vi "0xE6_Read_all_telemetry_data.vi"(7 "error in":errorcluster, 10 "paramUnicorn":T1={"conParam"={"ReadIntParam"=TRUE, "ReadDescrParam"=FALSE, "ReadFloatParam"=TRUE, "debug"=FALSE, "ReadJSON"=TRUE, "IP_address"="192.168.1.216", "N_attempts"=3, "type_con"=enum."TCP", "MB_address"=1, "VISA"="COM1", "connection ID"=refnum, "nameDevices"="", "timeout"=3000, "port"=2000, "type_version"="0F0C0001", "baud_rate"=115200, "VersionControl"=TRUE, "TCP_conn"=TRUE, "WindowSize"=700}, "Param"={"NumParam"={"NTelem"=201, "NInt"=16, "NFloat"=10, "NTable"=2}, "ParamInt"=[{"ID"="Режим работы", "Num"=0, "Name"="", "Type"="", "Enum"="", "Desc"="", "Unit"="", "Access"="", "FormatStr"="", "Min"=0, "Max"=0}, {"ID"="", "Num"=0, "Name"="", "Type"="", "Enum"="", "Desc"="", "Unit"="", "Access"="", "FormatStr"="", "Min"=0, "Max"=0}, {"ID"="", "Num"=0, "Name"="", "Type"="", "Enum"="", "Desc"="", "Unit"="", "Access"="", "FormatStr"="", "Min"=0, "Max"=0}, {"ID"="", "Num"=0, "Name"="", "Type"="", "Enum"="", "Desc"="", "Unit"="", "Access"="", "FormatStr"="", "Min"=0, "Max"=0}, {"ID"="", "Num"=0, "Name"="", "Type"="", "Enum"="", "Desc"="", "Unit"="", "Access"="", "FormatStr"="", "Min"=0, "Max"=0}, {"ID"="", "Num"=0, "Name"="", "Type"="", "Enum"="", "Desc"="", "Unit"="", "Access"="", "FormatStr"="", "Min"=0, "Max"=0}, {"ID"="ModeWork", "Num"=0, "Name"="", "Type"="", "Enum"="", "Desc"="", "Unit"="", "Access"="", "FormatStr"="", "Min"=0, "Max"=0}], "Telemetry"=[], "Table"=[], "ParamFloat"=[]}}) -> (0 "error out":errorcluster, 1 "Telemetry":sgl[](array[numeric]), 2 "TblTelemetry":string[][](array[string]), 3 "paramUnicorn 2":T1={"conParam"={"ReadIntParam"=TRUE, "ReadDescrParam"=FALSE, "ReadFloatParam"=TRUE, "debug"=FALSE, "ReadJSON"=TRUE, "IP_address"="192.168.1.216", "N_attempts"=3, "type_con"=enum."TCP", "MB_address"=1, "VISA"="COM1", "connection ID"=refnum, "nameDevices"="", "timeout"=3000, "port"=2000, "type_version"="0F0C0001", "baud_rate"=115200, "VersionControl"=TRUE, "TCP_conn"=TRUE, "WindowSize"=700}, "Param"={"NumParam"={"NTelem"=201, "NInt"=16, "NFloat"=10, "NTable"=2}, "ParamInt"=[{"ID"="Режим работы", "Num"=0, "Name"="", "Type"="", "Enum"="", "Desc"="", "Unit"="", "Access"="", "FormatStr"="", "Min"=0, "Max"=0}, {"ID"="", "Num"=0, "Name"="", "Type"="", "Enum"="", "Desc"="", "Unit"="", "Access"="", "FormatStr"="", "Min"=0, "Max"=0}, {"ID"="", "Num"=0, "Name"="", "Type"="", "Enum"="", "Desc"="", "Unit"="", "Access"="", "FormatStr"="", "Min"=0, "Max"=0}, {"ID"="", "Num"=0, "Name"="", "Type"="", "Enum"="", "Desc"="", "Unit"="", "Access"="", "FormatStr"="", "Min"=0, "Max"=0}, {"ID"="", "Num"=0, "Name"="", "Type"="", "Enum"="", "Desc"="", "Unit"="", "Access"="", "FormatStr"="", "Min"=0, "Max"=0}, {"ID"="", "Num"=0, "Name"="", "Type"="", "Enum"="", "Desc"="", "Unit"="", "Access"="", "FormatStr"="", "Min"=0, "Max"=0}, {"ID"="ModeWork", "Num"=0, "Name"="", "Type"="", "Enum"="", "Desc"="", "Unit"="", "Access"="", "FormatStr"="", "Min"=0, "Max"=0}], "Telemetry"=[], "Table"=[], "ParamFloat"=[]}})   [LabVIEW 2017, in "LV_Unicorn.lvlib"]
uses:
  LV_Unicorn.lvlib
  Control/unicorn_Param.ctl
  Control/unicorn_conn.ctl
  Control/unicorn_JSON.ctl
  Control/unicorn_ParamInt.ctl
  Control/unicorn_Telemetry.ctl
  Control/unicorn_Table.ctl
  Control/unicorn_ParamFloat.ctl
panel:
  out "String in":string
  out "String out":string
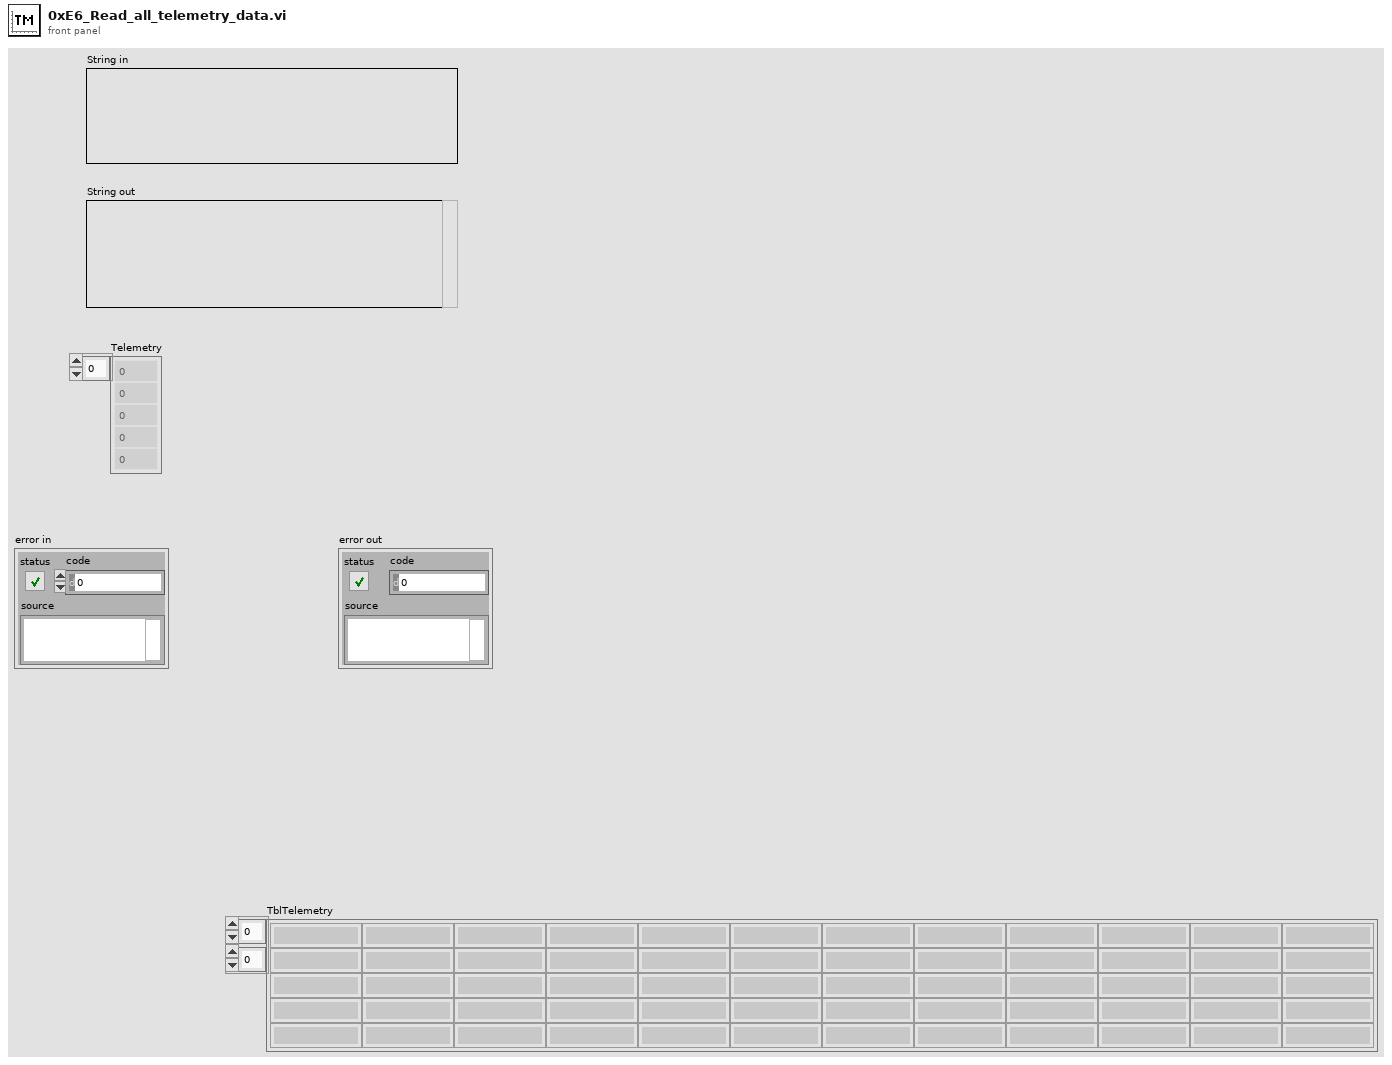
[diagram p1: front panel]
types:
  T1 = typedef "LV_Unicorn.lvlib/unicorn_Param.ctl" = cluster{"conParam":T2, "Param":T3}
  T2 = typedef "LV_Unicorn.lvlib/unicorn_conn.ctl" = cluster{"ReadIntParam":bool, "ReadDescrParam":bool, "ReadFloatParam":bool, "debug":bool, "ReadJSON":bool, "IP_address":string, "N_attempts":i32, "type_con":enum16{"Serial", "TCP"}, "MB_address":i32, "VISA":refnum<visa-resource-name>, "connection ID":refnum<k5>, "nameDevices":string, "timeout":i32, "port":u16, "type_version":string, "baud_rate":u32, "VersionControl":bool, "TCP_conn":bool, "WindowSize":i32}
  T3 = typedef "LV_Unicorn.lvlib/unicorn_JSON.ctl" = cluster{"NumParam":cluster{"NTelem":i32, "NInt":i32, "NFloat":i32, "NTable":i32}, "ParamInt":T4, "Telemetry":T5, "Table":T6, "ParamFloat":T7}
  T4 = typedef "LV_Unicorn.lvlib/unicorn_ParamInt.ctl" = cluster{"ID":string, "Num":i32, "Name":string, "Type":string, "Enum":string, "Desc":string, "Unit":string, "Access":string, "FormatStr":string, "Min":i32, "Max":i32}[]
  T5 = typedef "LV_Unicorn.lvlib/unicorn_Telemetry.ctl" = cluster{"ID":string, "Num":i32, "Name":string, "Desc":string, "Unit":string, "FormatStr":string, "Min":i32, "Max":i32}[]
  T6 = typedef "LV_Unicorn.lvlib/unicorn_Table.ctl" = cluster{"Num":i32, "Access":string, "ColumnCount":i32, "NeedParamPrepare":bool, "Columns":cluster{"Column":i32, "Desc":string, "Name":string}[], "DataType":string, "FormatStr":string, "ID":string, "Name":string, "RowCount":i32, "Rows":cluster{"Desc":string, "ID":string, "Max":i32, "Min":i32, "Name":string, "Row":i32, "Unit":string}[], "Type":string}[]
  T7 = typedef "LV_Unicorn.lvlib/unicorn_ParamFloat.ctl" = cluster{"ID":string, "Num":i32, "Name":string, "Type":string, "Enum":string, "Desc":string, "Unit":string, "Access":string, "FormatStr":string, "Min":sgl, "Max":sgl}[]
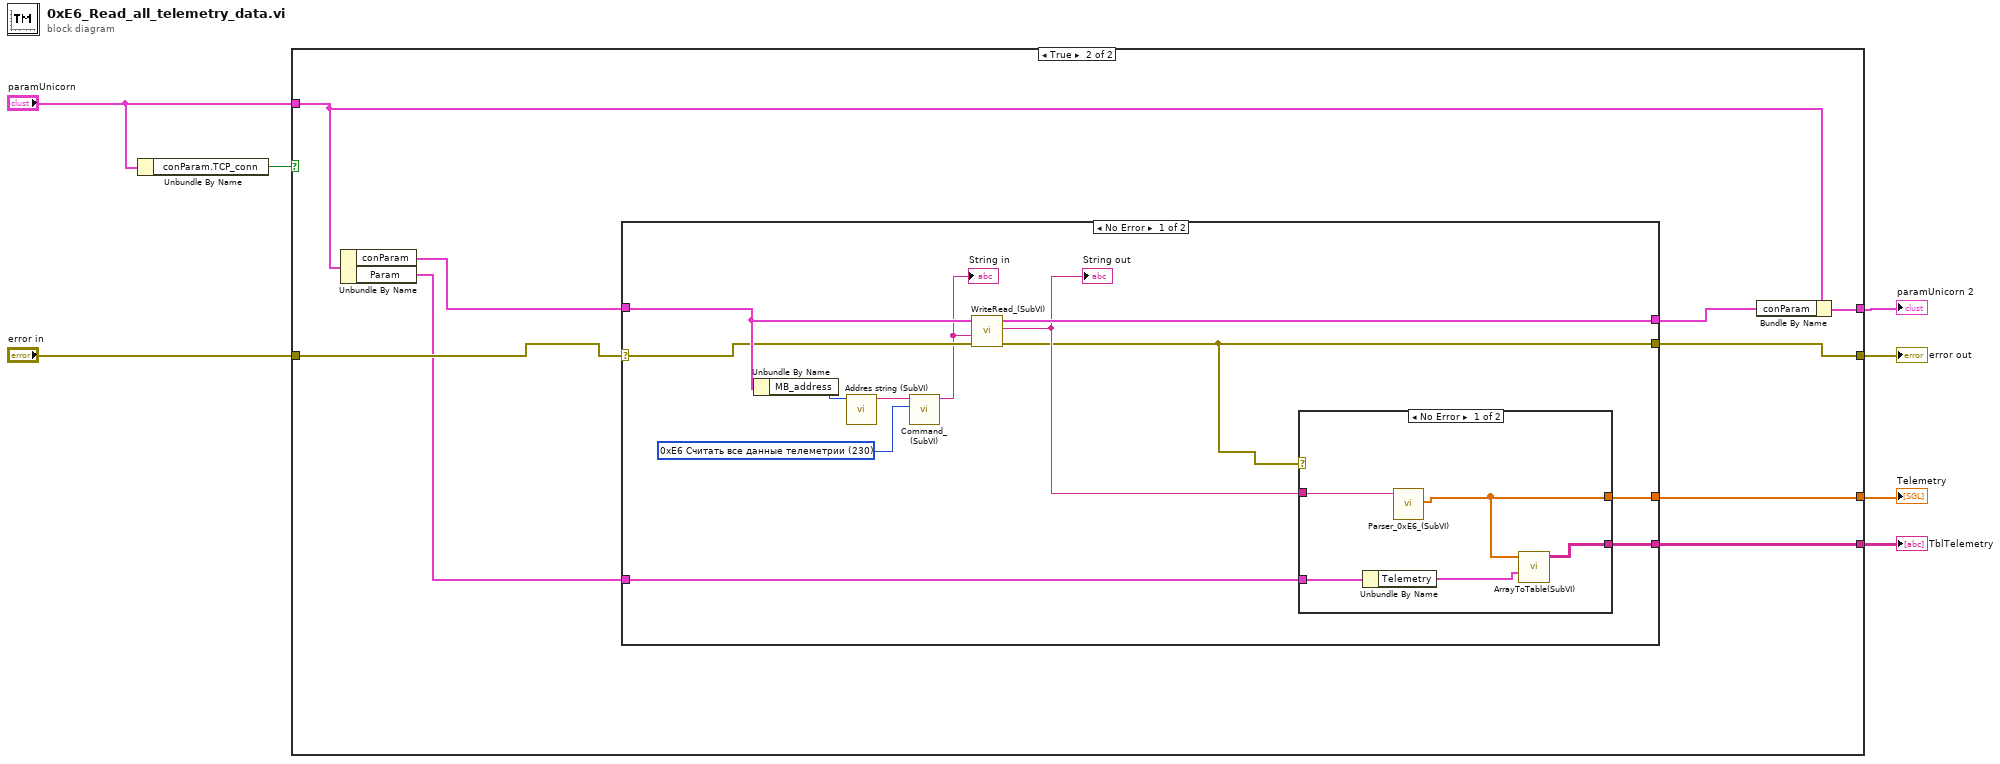
[diagram p0: block diagram]
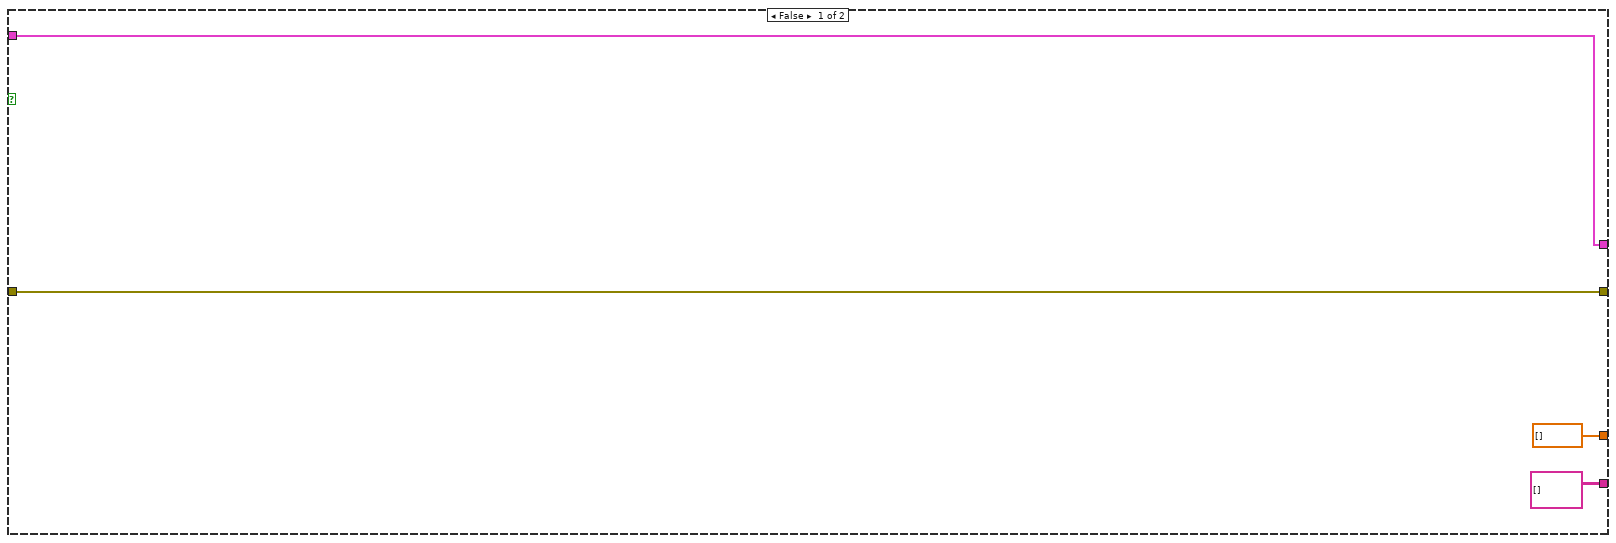
[diagram p2: hidden frame]
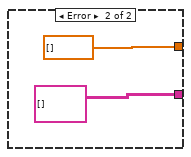
[diagram p3: hidden frame]
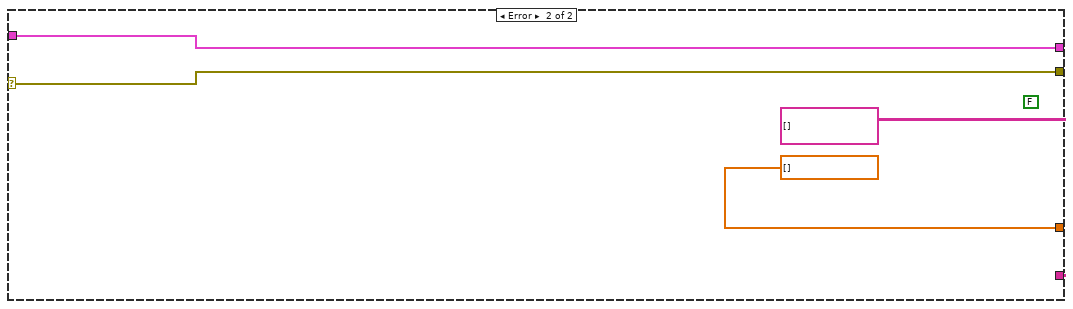
[diagram p4: hidden frame]
diagram:
  n1 = Unbundle By Name("paramUnicorn") -> ("conParam.TCP_conn"=w1:bool)
  n2 = case shown="True" w1 {
    tunnel: [sgl[] [] ("Array") w20] -> w7
    tunnel: "error in" -> [w10 w19]
    tunnel: [w10 w18] -> w5
    tunnel: [string[][] [] ("Таблица телеметрии") w17] -> w4
    tunnel: "paramUnicorn" -> [w11 w14]
    tunnel: [w11 w12] -> w3
    frame False {
    }
    frame True {
      n3 = Unbundle By Name(w14) -> ("conParam"=w16:T2, "Param"=w15:T3)
      n4 = case shown="No Error" w19 {
        selector: w19 -> [w26 w42]
        tunnel: [w32 sgl[] []] -> w20
        tunnel: w16 -> [w27 w43]
        tunnel: [w31 w43] -> w13
        tunnel: [w21 w42] -> w18
        tunnel: [w23 string[][] [] ("Таблица телеметрии")] -> w17
        tunnel: w15 -> [w22 _]
        frame No Error {
          w29 = u16 230 items=["0xE0 Запрос количества доступных параметров"=224, "0xE1 Записать один параметр типа float"=225, "0xE2 Записать один параметр типа int"=226, "0xE3 Считать один параметр телеметрии"=227, "0xE4 Записать все параметры типа float"=228, "0xE5 Записать все параметры типа int"=229, "0xE6 Считать все данные телеметрии"=230, "0xE7 Получить описание одного параметра типа float"=231, "0xE8 Получить описание одного параметра типа int"=232, "0xE9 Получить описание одного параметра телеметрии"=233, "0xEA Считать один параметр типа float"=234, "0xEB Считать один параметр типа int"=235, "0xEC Считать все параметры типа float"=236, "0xED Считать все параметры типа int"=237, "0xEE Считать считать фрагмент описания устройства в формате JSON"=238, "0x06 Записать UUID"=6, "0x07 Чтение UUID"=7, "0x45 Считывание параметров Flash памяти"=69, "0x43 Запись страницы Flash памяти"=67, "0x44 Чтения страницы Flash памяти"=68, "0x46 Получить описание Flash-памяти"=70, "0xFA Программный сброс"=250, "0xFB Изменение скорости интерфейса"=251, "0xFF Считывание типа и версии устройства"=255, "0x50 Запрос кол-ва табличных параметров"=80, "0x51 Запрос описания табличного параметра"=81, "0x52 Чтение данных табличного параметра"=82, "0x53 Запись данных табличного параметра"=83, "0x54 Подготовка табличного параметра"=84, "0x55 Запрос прогресса подготовки табличного параметра"=85, "0x56 Освобождение данных подготовленного табличного параметра"=86] ("Команда")
          n5 = Unbundle By Name(w27) -> ("MB_address"=w25:i32)
          n6 = call "Addres string (SubVI).vi"("Адрес"=w25) -> ("String"=w30:string)  [unwired: 10 in]
          n7 = call "Command_(SubVI).vi"("Команда"=w29, "String in"=w30) -> ("String out"=w24:string)  [unwired: 9 in]
          "String in" <- w24
          n8 = call "WriteRead_(SubVI).vi"("error in"=w26, "Запрос"=w24, "ParamIn"=w27) -> ("error out"=w21:errorcluster, "Ответ"=w28:string, "ParamOut"=w31:T2)  [unwired: 4 in, 2 out]
          "String out" <- w28
          n9 = case shown="No Error" w21 {
            tunnel: [w35 sgl[] [] ("Array")] -> w32
            tunnel: w28 -> [w37 _]
            tunnel: [w36 string[][] [] ("Таблица телеметрии")] -> w23
            tunnel: w22 -> [w34 _]
            frame No Error {
              n10 = Unbundle By Name(w34) -> ("Telemetry"=w33:T5)
              n11 = call "Parser_0xE6_(SubVI).vi"("String in"=w37) -> ("Array"=w35:sgl[])  [unwired: 9 in, 1 out]
              n12 = call "ArrayToTable(SubVI).vi"("Telemetry"=w33, "Data in"=w35) -> ("Table out"=w36:string[][])  [unwired: 9 in]
            }
            frame Error {
            }
          }
        }
        frame Error {
          (unwired) FALSE
        }
      }
      n13 = Bundle By Name(cluster=w14, "conParam"=w13) -> (w12:T1)
    }
  }
  "Telemetry" <- w7
  "error out" <- w5
  "TblTelemetry" <- w4
  "paramUnicorn 2" <- w3
